vi "bidirectional PC network streamI.vi"(8 "error in":errorcluster, 9 "SEND":bool, 10 "Message To Send":T1={"Command"="Cmd From PC", "Arguments"=variant(string "Arguments are variants. Wire anything!"), " Msg Id"=0}, 11 "Settings":T2={"My Name"="PC", "Remote IP Address"="localhost", "Remote Name"="RT"}) -> (0 "error out":errorcluster, 2 "Incoming Messages":T1[](array[typedef]))   [LabVIEW 2020]
doc: "Provides a basic example of a PC user interface that uses network streams to connect to a remote system.JKI Network Streams Connection 1.1.1.15\nJavier Ruiz - JKI\nCopyright (c) 2020, JKI\n\nThis library is provided \"AS IS\" ,WITHOUT WARRANTIES OR CONDITIONS OF ANY KIND, either express or implied."
uses:
  <vilib>/addons/_JKI.lib/Network_Streams_Connection.llb/NetworkCommand--Cluster.ctl
  <vilib>/addons/_JKI.lib/Network_Streams_Connection.llb/PublicSettings.ctl
  <vilib>/addons/_JKI.lib/Network_Streams_Connection.llb/NetworkConnection.lvclass/NetworkConnection.ctl
  <vilib>/addons/_JKI.lib/Network_Streams_Connection.llb/NetworkConnection.lvclass
panel:
  in  "Fast timeout(ms)":i32=100
  in  "Slow timeout(ms)":i32=500
  in  "Stop":bool
  out "Timed Out?":bool
  out "Connected?":bool
  # "JKI Network Stream 2-Way Communication Example\nPC Endpoint"
  # "Instructions: \n- Configure the settings below before running the VI: \n   IP Address is only needed on one end \n- Run the other endpoint.\n- If settings are the same the code will reconnect automatically\n- Type a Cmd Name and Click Send\n- Send from the other endpoint to see messages arrive here"
  # "*Arguments are variants\nso you can wire anything!"
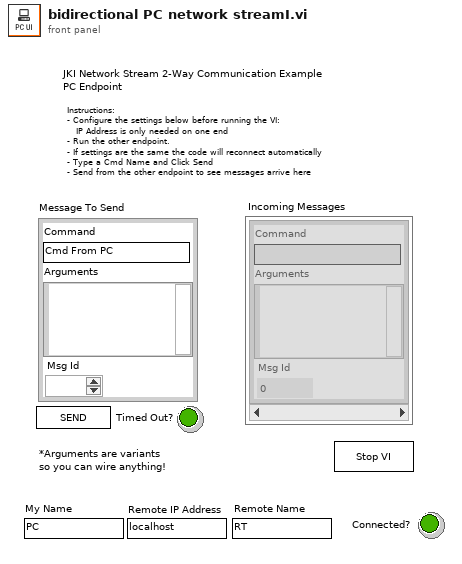
[diagram p1: front panel]
types:
  T1 = typedef "NetworkConnection.lvclass/NetworkCommand--Cluster.ctl" = cluster{"Command":string, "Arguments":variant, " Msg Id":i32}
  T2 = typedef "NetworkConnection.lvclass/PublicSettings.ctl" = cluster{"My Name":string, "Remote IP Address":string, "Remote Name":string}
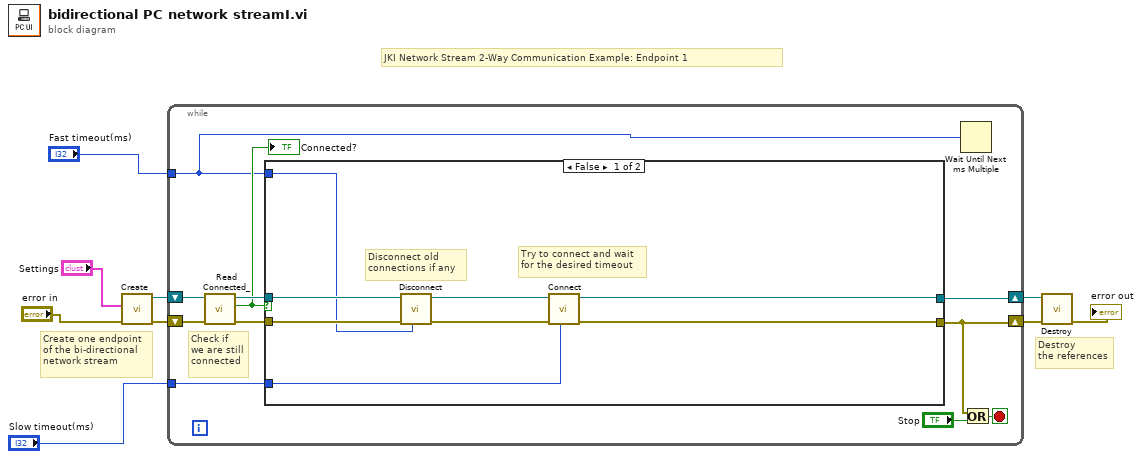
[diagram p0: block diagram]
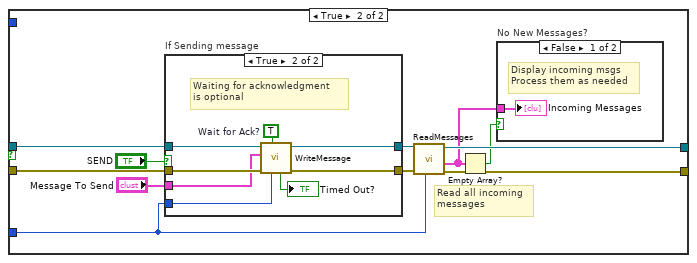
[diagram p2: hidden frame]
diagram:
  # "Destroy\nthe references"
  # "Create one endpoint\nof the bi-directional\nnetwork stream"
  # "JKI Network Stream 2-Way Communication Example: Endpoint 1"
  n1 = call <vilib>:"Create.vi"("error in (no error)"="error in", "Settings"="Settings") -> ("error out"=w6:errorcluster, "NetworkConnection out"=w8:refnum<class "NetworkConnection.lvclass">)  [unwired: 8 in]
  n2 = while {
    shift-right: [w16] -> w7
    shift-left: w8 -> [w20]
    shift-right: [w13] -> w5
    shift-left: w6 -> [w19]
    tunnel: "Slow timeout(ms)" -> [w11]
    tunnel: "Fast timeout(ms)" -> [w10]
    stop <- w12 stop-if-true
    # "Check if\nwe are still\nconnected"
    n3 = call <vilib>:"Read Connected_.vi"("error in (no error)"=w19, "NetworkConnection in"=w20) -> ("error out"=w18:errorcluster, "Connected?"=w15:bool, "NetworkConnection out"=w17:refnum<class "NetworkConnection.lvclass">)  [unwired: 7 in]
    "Connected?" <- w15
    n4 = case shown="False" w15 {
      tunnel: w18 -> [w24 w35]
      tunnel: w17 -> [w26 w36]
      tunnel: [w27 w39] -> w16
      tunnel: [w28 w38] -> w13
      tunnel: w11 -> [w22 w29]
      tunnel: w10 -> [w21 _]
      frame False {
        # "Try to connect and wait\nfor the desired timeout"
        # "Disconnect old\nconnections if any"
        n5 = call <vilib>:"Disconnect.vi"("Timeout ms (1000)"=w21, "error in (no error)"=w24, "NetworkConnection in"=w26) -> ("error out"=w23:errorcluster, "NetworkConnection out"=w25:refnum<class "NetworkConnection.lvclass">)  [unwired: 7 in]
        n6 = call <vilib>:"Connect.vi"("Timeout(ms)"=w22, "error in (no error)"=w23, "NetworkConnection in"=w25) -> ("error out"=w28:errorcluster, "NetworkConnection out"=w27:refnum<class "NetworkConnection.lvclass">)  [unwired: 6 in, 1 out]
      }
      frame True {
        # "Read all incoming\nmessages"
        n7 = case "If Sending message" shown="True" "SEND" {
          tunnel: w36 -> [w42 w50]
          tunnel: w35 -> [w41 w49]
          tunnel: "Message To Send" -> [_ w48]
          tunnel: w29 -> [_ w47]
          tunnel: [w41 w44] -> w33
          tunnel: [w42 w43] -> w32
          frame False {
          }
          frame True {
            w46 = TRUE  # Wait for Ack?
            # "Waiting for acknowledgment\nis optional"
            n8 = call <vilib>:"WriteMessage.vi"("Timeout(ms)"=w47, "Wait for Ack? (false)"=w46, "error in (no error)"=w49, "Message"=w48, "NetworkConnection in"=w50) -> ("error out"=w44:errorcluster, "NetworkConnection out"=w43:refnum<class "NetworkConnection.lvclass">, "Timed Out?"=→"Timed Out?":bool)  [unwired: 3 in, 1 out]
          }
        }
        n9 = call <vilib>:"ReadMessages.vi"("Timeout(ms)"=w29, "error in (no error)"=w33, "NetworkConnection in"=w32) -> ("error out"=w38:errorcluster, "Messages"=w30:T1[], "NetworkConnection out"=w39:refnum<class "NetworkConnection.lvclass">)  [unwired: 4 in, 2 out]
        n10 = Empty Array?(array=w30) -> (empty?=w31:bool)
        n11 = case "No New Messages?" shown="False" w31 {
          tunnel: w30 -> [w40 _]
          frame False {
            # "Display incoming msgs\nProcess them as needed"
            "Incoming Messages" <- w40
          }
          frame True {
          }
        }
      }
    }
    n12 = Wait Until Next ms Multiple(millisecond multiple=w10) -> ()  [unwired: 1 out]
    n13 = Or(x=w13, y="Stop") -> (x .or. y?=w12:bool)
  }
  n14 = call <vilib>:"Destroy.vi"("error in (no error)"=w5, "NetworkConnection in"=w7) -> ("error out"=→"error out":errorcluster)  [unwired: 8 in, 1 out]
